vi "current monitor.vi"() -> ()   [LabVIEW 2010]
uses:
  <vilib>/Utility/file.llb/Write To Spreadsheet File (DBL).vi
  <userlib>/Nanonis Prog Interface V5/Nanonis Prog Interface.lvlib
panel:
  in  "Convert to nm/s?":bool caption="Spectrum Analyzer 2"
  out "Spectrum Analyzer 2":cluster{"f0":dbl, "df":dbl, "values":dbl[]}(graph)
  in  "Spectrum Analyzer2":bool caption="Spectrum Analyzer 2"
  out "error out":errorcluster
  in  "Path":path
  out "Spectrum Analyzer":cluster{"f0":dbl, "df":dbl, "values":dbl[]}(graph)
  out "Current (A)":sgl format="%#_6p"
  out "Current":cluster{"Current (A)":dbl, dbl}[](graph)
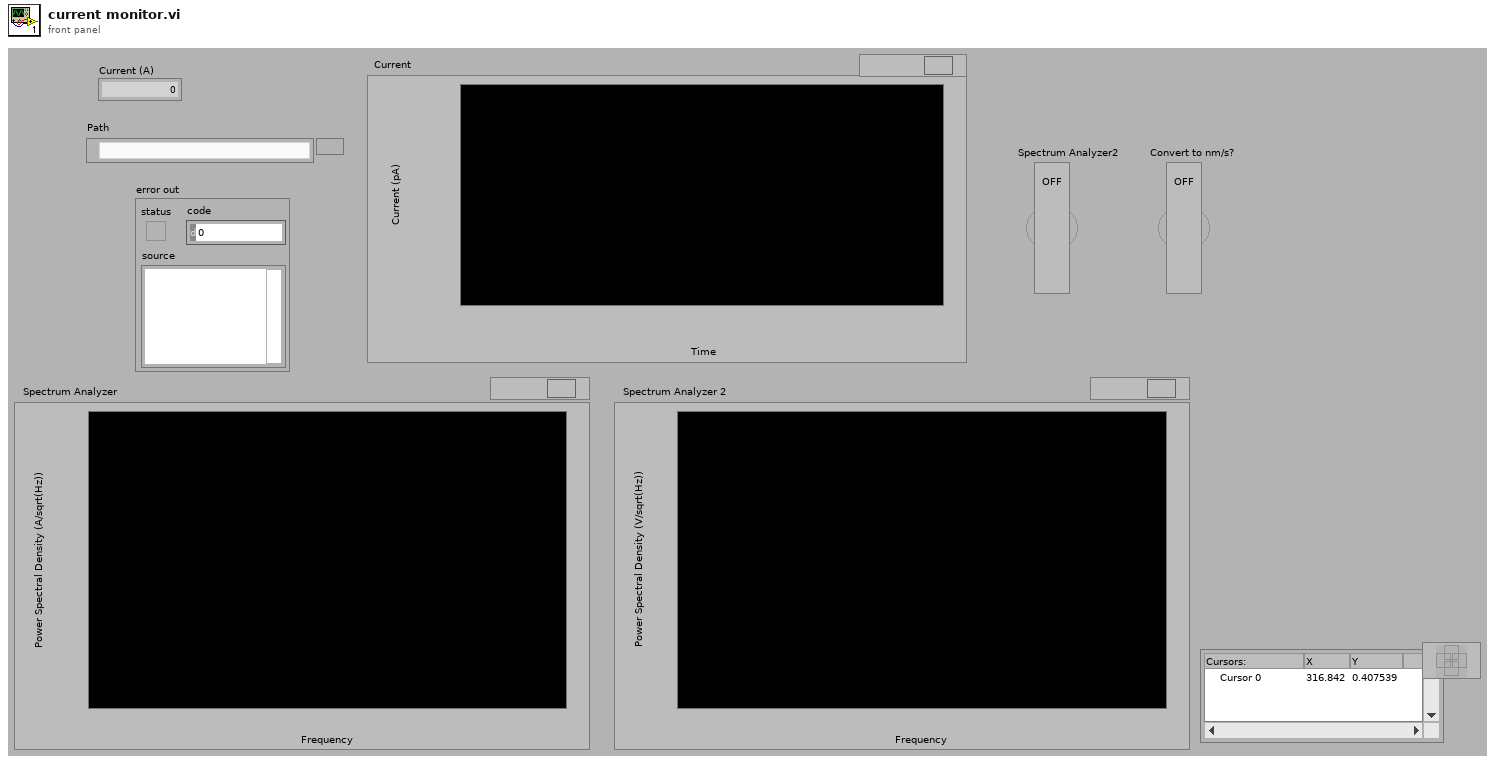
[diagram p1: front panel]
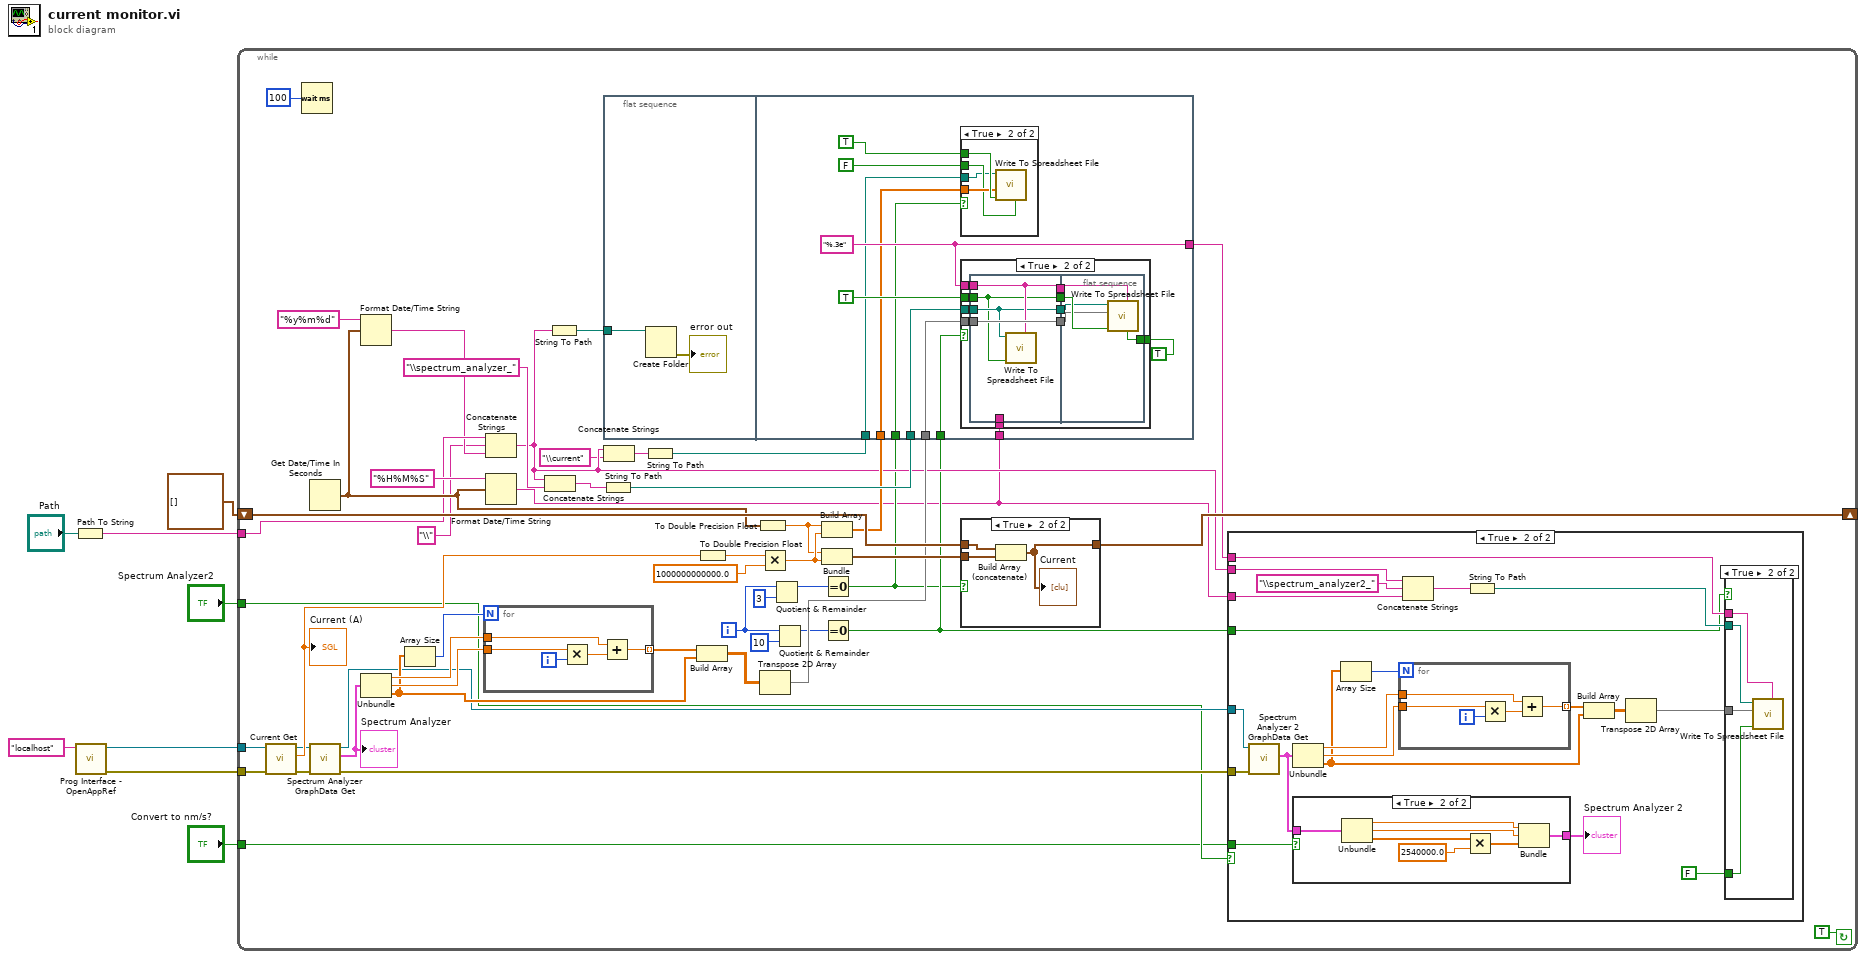
[diagram p0: block diagram]
diagram:
  n1 = Path To String(path="Path") -> (string=w3:string)
  n2 = call <userlib>:"Prog Interface - OpenAppRef.vi"("Machine name (local machine IP)"="localhost" ("machine name (localhost)")) -> ("Error out"=w7:errorcluster, "Application reference"=w8:refnum<vi>)  [unwired: 5 in]
  n3 = while {
    tunnel: w8 -> [w57]
    tunnel: w7 -> [w56]
    shift-right: [w53] -> _
    shift-left: cluster{dbl, dbl}[] [] -> [w54]
    tunnel: w3 -> [w41]
    tunnel: "Spectrum Analyzer2" -> [w26]
    tunnel: "Convert to nm/s?" -> [w24]
    i -> [w11]
    stop <- TRUE continue-if-true
    n4 = call <userlib>:"Current Get.vi"("Error in (no error)"=w56, "Application ref in"=w57) -> ("Error out"=w48:errorcluster, "Current (A)"=w52:sgl, "Application ref out"=w49:refnum<vi>)  [unwired: 5 in]
    "Current (A)" <- w52
    n5 = Wait (ms)(milliseconds to wait=u32 100) -> ()  [unwired: 1 out]
    n6 = Get Date/Time In Seconds() -> (seconds since 1Jan1904=w42:timestamp)
    n7 = call <userlib>:"Spectrum Analyzer GraphData Get.vi"("Error in (no error)"=w48, "Application ref in"=w49) -> ("Error out"=w27:errorcluster, "FFT data"=w46:cluster{"f0":dbl, "df":dbl, "values":dbl[]}, "Application ref out"=w28:refnum<vi>)  [unwired: 7 in]
    "Spectrum Analyzer" <- w46
    n8 = Format Date/Time String(time format string (%c)="%y%m%d", seconds (now)=w42) -> (date/time string=w39:string)  [unwired: 1 in]
    n9 = Unbundle(w46) -> ("f0"=w34:dbl, "df"=w33:dbl, "values"=w31:dbl[])
    n10 = Array Size(array=w31) -> (size(s)=w35:i32)
    n11 = for {
      N: w35 -> [_]
      tunnel: w34 -> [w104]
      tunnel: w33 -> [w101]
      tunnel: [w100] -> w32 mode=indexing
      i -> [w102]
      n12 = Multiply(x=w101, y=w102) -> (x*y=w103:dbl)
      n13 = Add(x=w104, y=w103) -> (x+y=w100:dbl)
    }
    n14 = Concatenate Strings(w41, "\\" ("string"), w39) -> (w22:string)
    n15 = Format Date/Time String(time format string (%c)="%H%M%S", seconds (now)=w42) -> (date/time string=w9:string)  [unwired: 1 in]
    n16 = Concatenate Strings(w22, "\\spectrum_analyzer_" ("string")) -> (w36:string)
    n17 = String To Path(string=w22) -> (path=w40:path)
    n18 = String To Path(string=w36) -> (path=w44:path)
    n19 = flat-sequence {
      tunnel: w40 -> [w106]
      tunnel: w44 -> [w111]
      tunnel: w29 -> [w112]
      tunnel: [w117] -> w25
      tunnel: w23 -> [w115]
      tunnel: w19 -> [w113]
      tunnel: w14 -> [w110]
      tunnel: w10 -> [w109]
      tunnel: w9 -> [w107]
      frame #0 {
        n20 = Create Folder(path (use dialog)=w106) -> (error out=→"error out":errorcluster)  [unwired: 2 in, 2 out]
      }
      frame #1 {
        w117 = "%.3e" ("format (%.3f)")
        n21 = case shown="True" w109 {
          tunnel: TRUE ("append to file? (new file:F)") -> [_ w122]
          tunnel: w115 -> [_ w121]
          tunnel: FALSE ("transpose? (no:F)") -> [_ w120]
          tunnel: w113 -> [_ w119]
          frame False {
          }
          frame True {
            n22 = call-poly <vilib>:"Write To Spreadsheet File.vi"("transpose? (no:F)"=w120, "append to file? (new file:F)"=w122, "1D data"=w121, "file path (dialog if empty)"=w119) -> ()  [unwired: 4 in, 1 out]
          }
        }
        n23 = case shown="True" w110 {
          tunnel: TRUE ("append to file? (new file:F)") -> [_ w132]
          tunnel: w117 -> [_ w131]
          tunnel: w112 -> [_ w130]
          tunnel: w111 -> [_ w129]
          tunnel: TRUE -> [_ w128]
          tunnel: w107 -> [_ w123]
          frame False {
          }
          frame True {
            n24 = flat-sequence {
              tunnel: w129 -> [w134]
              tunnel: w130 -> [w136]
              tunnel: w131 -> [w135]
              tunnel: w132 -> [w133]
              tunnel: [w133] -> w127
              tunnel: [w135] -> w126
              tunnel: [w136] -> w125
              tunnel: [w134] -> w124
              tunnel: w123 -> [_]
              tunnel: w128 -> [w137]
              tunnel: w127 -> [w141]
              tunnel: w126 -> [w140]
              tunnel: w125 -> [w139]
              tunnel: w124 -> [w138]
              frame #0 {
                n25 = call-poly <vilib>:"Write To Spreadsheet File.vi"("format (%.3f)"=w135, "append to file? (new file:F)"=w133, "file path (dialog if empty)"=w134) -> ()  [unwired: 5 in, 1 out]
              }
              frame #1 {
                n26 = call-poly <vilib>:"Write To Spreadsheet File.vi"("transpose? (no:F)"=w137, "format (%.3f)"=w140, "append to file? (new file:F)"=w141, "2D data"=w139, "file path (dialog if empty)"=w138) -> ()  [unwired: 3 in, 1 out]
              }
            }
          }
        }
      }
    }
    n27 = Concatenate Strings(w22, "\\current" ("string")) -> (w20:string)
    n28 = String To Path(string=w20) -> (path=w19:path)
    n29 = Build Array(w32, w31) -> (w30:dbl[][])
    n30 = To Double Precision Float(number=w52) -> (double precision float=w51:dbl)
    n31 = To Double Precision Float(number=w42) -> (double precision float=w17:dbl)
    n32 = Multiply(x=w51, y=1000000000000.0) -> (x*y=w18:dbl)
    n33 = Transpose 2D Array(2D array=w30) -> (transposed array=w29:dbl[][])
    n34 = Quotient & Remainder(x=w11, y=3) -> (x-y*floor(x/y)=w12:i32)  [unwired: 1 out]
    n35 = Quotient & Remainder(x=w11, y=10) -> (x-y*floor(x/y)=w15:i32)  [unwired: 1 out]
    n36 = Build Array(w17, w18) -> (w23:dbl[])
    n37 = Bundle(w17, w18) -> (w55:cluster{dbl, dbl})  [unwired: 1 in]
    n38 = Equal To 0?(x=w12) -> (x = 0?=w10:bool)
    n39 = Equal To 0?(x=w15) -> (x = 0?=w14:bool)
    n40 = case shown="True" w10 {
      tunnel: w55 -> [_ w62]
      tunnel: w54 -> [w59 w61]
      tunnel: [w59 w60] -> w53
      frame False {
      }
      frame True {
        n41 = Build Array (concatenate)(w61, w62) -> (w60:cluster{dbl, dbl}[])
        "Current" <- w60
      }
    }
    n42 = case shown="True" w26 {
      tunnel: w28 -> [_ w82]
      tunnel: w27 -> [_ w81]
      tunnel: w22 -> [_ w72]
      tunnel: w9 -> [_ w71]
      tunnel: w25 -> [_ w67]
      tunnel: w24 -> [_ w64]
      tunnel: w14 -> [_ w63]
      frame False {
      }
      frame True {
        n43 = call <userlib>:"Spectrum Analyzer 2 GraphData Get.vi"("Error in (no error)"=w81, "Application ref in"=w82) -> ("FFT data"=w66:cluster{"f0":dbl, "df":dbl, "values":dbl[]})  [unwired: 7 in, 2 out]
        n44 = Unbundle(w66) -> ("f0"=w79:dbl, "df"=w78:dbl, "values"=w76:dbl[])
        n45 = case shown="True" w64 {
          tunnel: w66 -> [w87 w94]
          tunnel: [w87 w93] -> w65
          frame False {
          }
          frame True {
            n46 = Unbundle(w94) -> ("f0"=w92:dbl, "df"=w91:dbl, "values"=w90:dbl[])
            n47 = Multiply(x=w90, y=2540000.0) -> (x*y=w89:dbl[])
            n48 = Bundle("f0"=w92, "df"=w91, w89) -> (w93:cluster{"f0":dbl, "df":dbl, dbl[]})  [unwired: 1 in]
          }
        }
        "Spectrum Analyzer 2" <- w65
        n49 = Array Size(array=w76) -> (size(s)=w80:i32)
        n50 = for {
          N: w80 -> [_]
          tunnel: w79 -> [w99]
          tunnel: w78 -> [w96]
          tunnel: [w95] -> w75 mode=indexing
          i -> [w97]
          n51 = Multiply(x=w96, y=w97) -> (x*y=w98:dbl)
          n52 = Add(x=w99, y=w98) -> (x+y=w95:dbl)
        }
        n53 = Concatenate Strings(w72, "\\spectrum_analyzer2_" ("string"), w71) -> (w68:string)
        n54 = String To Path(string=w68) -> (path=w69:path)
        n55 = Build Array(w75, w76) -> (w77:dbl[][])
        n56 = Transpose 2D Array(2D array=w77) -> (transposed array=w73:dbl[][])
        n57 = case shown="True" w63 {
          tunnel: FALSE ("append to file? (new file:F)") -> [_ w86]
          tunnel: w73 -> [_ w85]
          tunnel: w69 -> [_ w84]
          tunnel: w67 -> [_ w83]
          frame False {
          }
          frame True {
            n58 = call-poly <vilib>:"Write To Spreadsheet File.vi"("format (%.3f)"=w83, "append to file? (new file:F)"=w86, "2D data"=w85, "file path (dialog if empty)"=w84) -> ()  [unwired: 4 in, 1 out]
          }
        }
      }
    }
  }
